vi "initialise.vi"(8 "error in (no error)":errorcluster, 11 "DL090602SutterMP285Stage in":refnum<class "StageDL090602SutterMP285.lvclass">) -> (0 "error out":errorcluster, 3 "DL090602SutterMP285Stage out":refnum<class "StageDL090602SutterMP285.lvclass">)   [LabVIEW 2010, in "StageDL090602SutterMP285.lvclass"]
doc: "The dynamic dispatch-version of this VI initalises the plug-in object by allocating and initalising any dynamic resources need."
uses:
  StageDL090602SutterMP285.lvclass
  StageDL090409Scaffold/StageDL090409Scaffold/StageDL090409Scaffold.lvclass
  StageDL090602SutterMP285.lvclass/StageDL090602SutterMP285.ctl
panel:
  in  "timeout (ms)":u32=3000
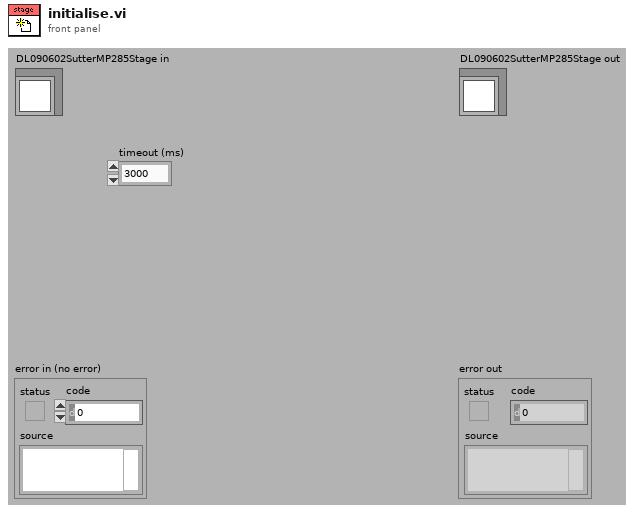
[diagram p1: front panel]
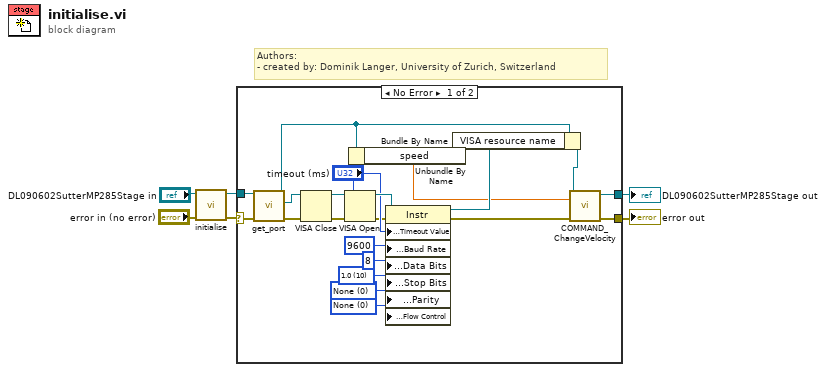
[diagram p0: block diagram]
diagram:
  # "Authors: \n- created by: Dominik Langer, University of Zurich, Switzerland"
  n1 = call-parent "initialise.vi"("error in (no error)"="error in (no error)", "GenericPlugin in"="DL090602SutterMP285Stage in") -> ("error out"=w4:errorcluster, "GenericPlugin out"=w3:refnum<class "StageDL090602SutterMP285.lvclass">)  [unwired: 8 out]
  n2 = case shown="No Error" w4 {
    selector: w4 -> [w26 w28]
    tunnel: w3 -> [w25 w27]
    tunnel: [w13 w28] -> w2
    tunnel: [w12 w27] -> w1
    frame No Error {
      w21 = u16 0 items=["None", "XON/XOFF", "RTS/CTS", "XON/XOFF & RTS/CTS", "DTR/DSR", "XON/XOFF & DTR/DSR"] ("Serial Settings:Flow Control")
      w20 = u16 0 items=["None", "Odd", "Even", "Mark", "Space"] ("Serial Settings:Parity")
      w19 = u16 10 items=["1.0"=10, "1.5"=15, "2.0"=20] ("Serial Settings:Stop Bits")
      n3 = call-dynamic "get_port.vi"("error in (no error)"=w26, "DL090602SutterMP285Stage in"=w25) -> ("error out"=w16:errorcluster, "serial port"=w14:refnum<visa-resource-name>, "DL090602SutterMP285Stage out"=w8:refnum<class "StageDL090602SutterMP285.lvclass">)  [unwired: 7 out]
      n4 = VISA Close(VISA resource name=w14, error in (no error)=w16) -> (error out=w15:errorcluster)
      n5 = VISA Open(timeout (0)="timeout (ms)", error in (no error)=w15, VISA resource name=w14) -> (VISA resource name=w24:refnum<visa-resource-name>, error out=w22:errorcluster)  [unwired: 2 out]
      n6 = Unbundle By Name(w8) -> ("speed"=w7:dbl[unit])
      n7 = property on="Property Node" class="Instr"(reference=w24, error in=w22, "General Settings:Timeout Value"="timeout (ms)", "Serial Settings:Baud Rate"=u32 9600, "Serial Settings:Data Bits"=u16 8, "Serial Settings:Stop Bits"=w19, "Serial Settings:Parity"=w20, "Serial Settings:Flow Control"=w21) -> (reference out=w9:refnum<visa-resource-name>, error out=w10:errorcluster)
      n8 = Bundle By Name(cluster=w8, "VISA resource name"=w9) -> (w11:refnum<class "StageDL090602SutterMP285.lvclass">)
      n9 = call-dynamic "COMMAND_ChangeVelocity.vi"("error in (no error)"=w10, "velocity"=w7, "StageDL090602SutterMP285 in"=w11) -> ("error out"=w13:errorcluster, "StageDL090602SutterMP285 out"=w12:refnum<class "StageDL090602SutterMP285.lvclass">)  [unwired: 7 in]
    }
    frame Error {
    }
  }
  "error out" <- w2
  "DL090602SutterMP285Stage out" <- w1
